vi "Set Common Pameters.vi"(6 "diameter abort (mm)":dbl, 7 "time delay (sec)":dbl=2.0, 8 "error in (no error)":errorcluster, 9 "sample rate (hz)":dbl, 10 "test time (sec)":dbl, 11 "IA Test Parameters in":refnum<class "IA Test Parameters.lvclass">) -> (0 "error out":errorcluster, 3 "IA Test Parameters out":refnum<class "IA Test Parameters.lvclass">)   [LabVIEW 2020, in "IA Test Parameters.lvclass"]
uses:
  IA Test Parameters.lvclass
  IA Test Parameters.lvclass/IA Test Parameters.ctl
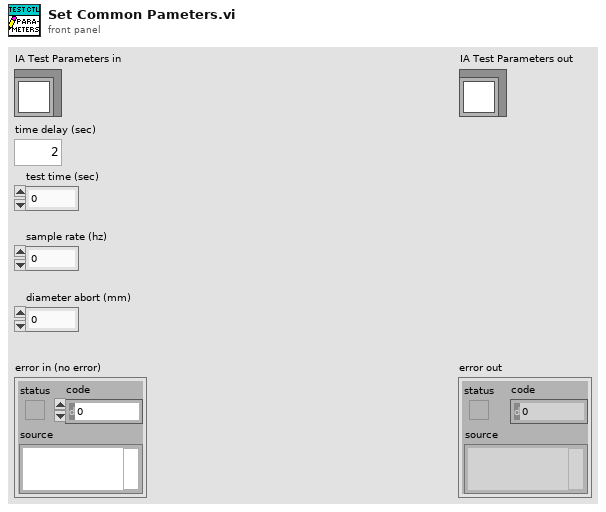
[diagram p1: front panel]
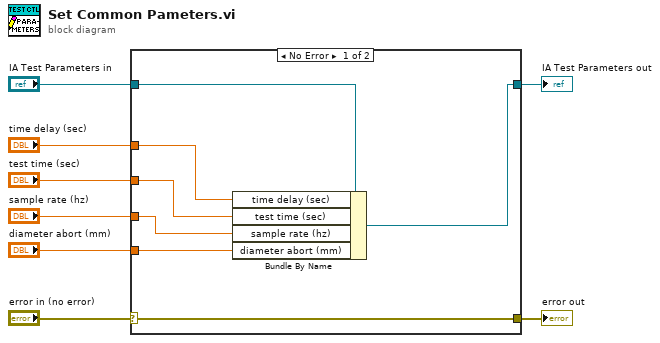
[diagram p0: block diagram]
diagram:
  n1 = case shown="No Error" "error in (no error)" {
    selector: "error in (no error)" -> [w15 w16]
    tunnel: [w15 w16] -> w7
    tunnel: [w13 w17] -> w5
    tunnel: "IA Test Parameters in" -> [w14 w17]
    tunnel: "time delay (sec)" -> [w12 _]
    tunnel: "test time (sec)" -> [w11 _]
    tunnel: "sample rate (hz)" -> [w10 _]
    tunnel: "diameter abort (mm)" -> [w9 _]
    frame No Error {
      n2 = Bundle By Name(cluster=w14, "time delay (sec)"=w12, "test time (sec)"=w11, "sample rate (hz)"=w10, "diameter abort (mm)"=w9) -> (w13:refnum<class "IA Test Parameters.lvclass">)
    }
    frame Error {
    }
  }
  "error out" <- w7
  "IA Test Parameters out" <- w5
